vi "Read G08 Settings.vi"(8 "error in (no error)":errorcluster, 11 "BME_DG_G08 in":refnum<class "BME_DG_G08.lvclass">) -> (0 "error out":errorcluster, 2 "SG08_Settings":T1={"Gate Terminate"=TRUE, "Gate Level"=1.0, "Gate Delay (µs)"=0.0, "StepBackTime (µs)"=0.0, "Burst Counter"=0, "Trigger Divider"=1, "Trigger Multiplier"=4} {"StepBackTime (µs)" min=0.0 format="%.6f"; "Gate Delay (µs)" format="%.3f"; "Gate Level" min=-2.5 max=2.5 format="%.3g"}, 3 "BME_DG_G08 out":refnum<class "BME_DG_G08.lvclass">)   [LabVIEW 2009, in "POLARIS BME DG.lvlib" / "BME_DG_G08.lvclass"]
uses:
  BME_DG_G08.lvclass
  LV-BME Interface/SG08_Settings.ctl
  BME_DG_G08.lvclass/BME_DG_G08.ctl
  POLARIS BME DG.lvlib
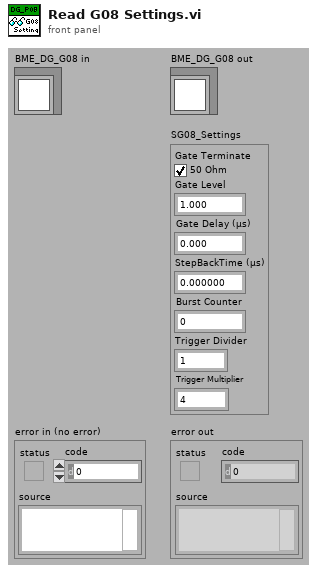
[diagram p1: front panel]
types:
  T1 = typedef "POLARIS BME DG.lvlib/SG08_Settings.ctl" = cluster{"Gate Terminate":bool, "Gate Level":dbl, "Gate Delay (µs)":dbl, "StepBackTime (µs)":dbl, "Burst Counter":u32, "Trigger Divider":u32, "Trigger Multiplier":u32}
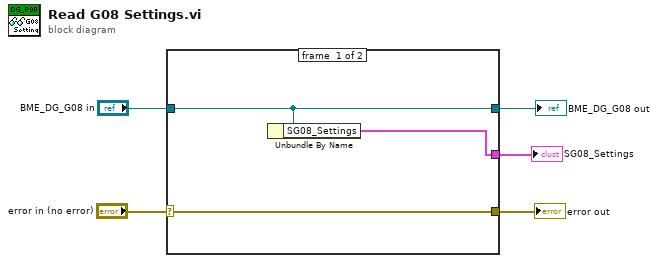
[diagram p0: block diagram]
diagram:
  n1 = case shown="No Error" "error in (no error)" {
    selector: "error in (no error)" -> [w8 w10]
    tunnel: [w8 w10] -> w4
    tunnel: [w7 w9] -> w2
    tunnel: "BME_DG_G08 in" -> [w7 w9]
    tunnel: [w6 _] -> w1
    frame #0 {
      n2 = Unbundle By Name(w7) -> ("SG08_Settings"=w6:T1)
    }
    frame #1 {
    }
  }
  "error out" <- w4
  "BME_DG_G08 out" <- w2
  "SG08_Settings" <- w1
